vi "editTest.vi"(8 "error in (no error)":errorcluster, 11 "TestInterface in":refnum<class "TestInterface.lvclass">) -> (0 "error out":errorcluster, 3 "TestInterface out":refnum<class "TestInterface.lvclass">)   [LabVIEW 2013, in "TestInterface.lvclass"]
uses:
  Tests/TestInterface/TestInterface.lvclass
panel:
  in  "Cancel Button":bool
  in  "OK Button":bool
  in  "Parameters":string[][](table)
  in  "wait":u32[](array[numeric])
  in  "timings":i32[](array[numeric])
  in  "response":bool[](array[boolean])
  in  "name":string
  in  "Commandlist":string
  in  "Command regex":string[](array[string])
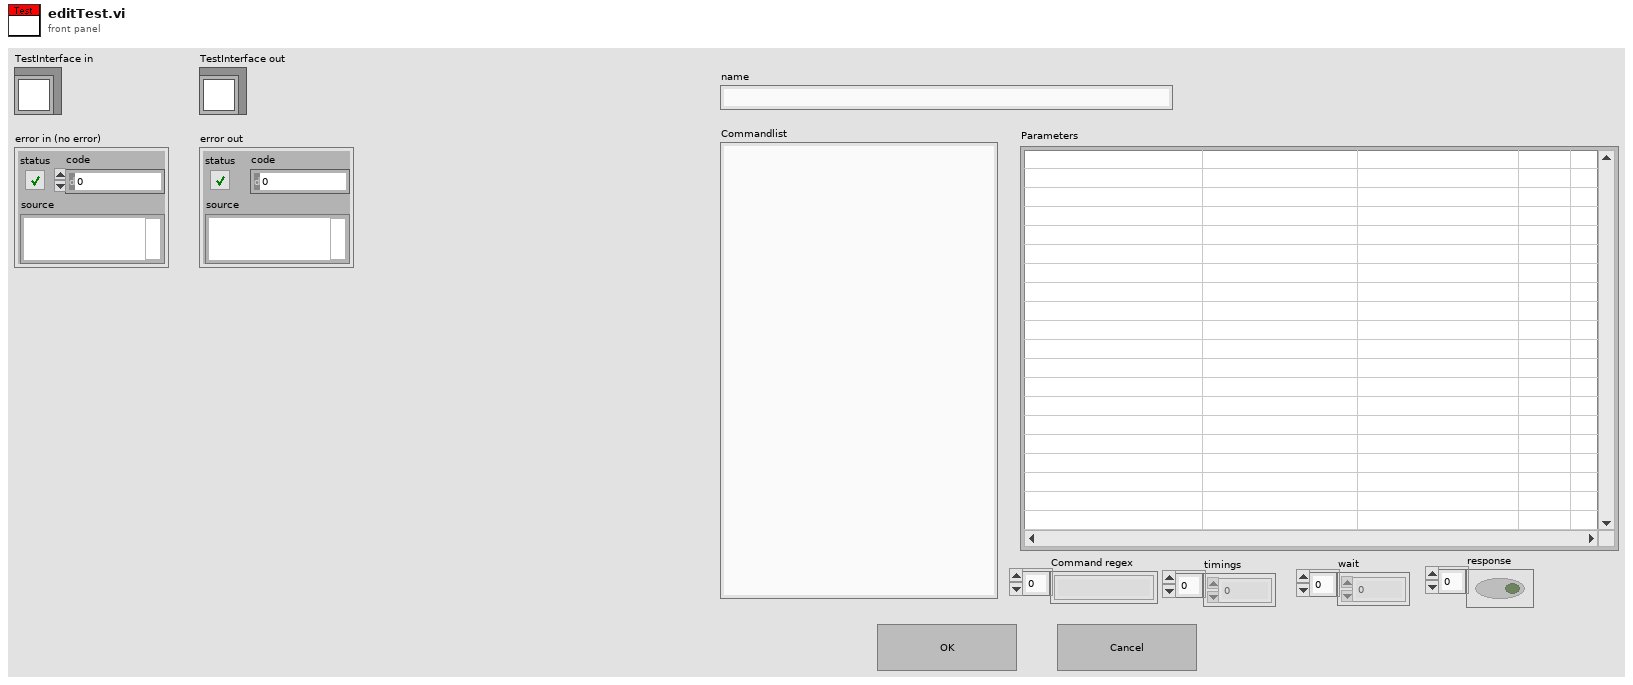
[diagram p1: front panel]
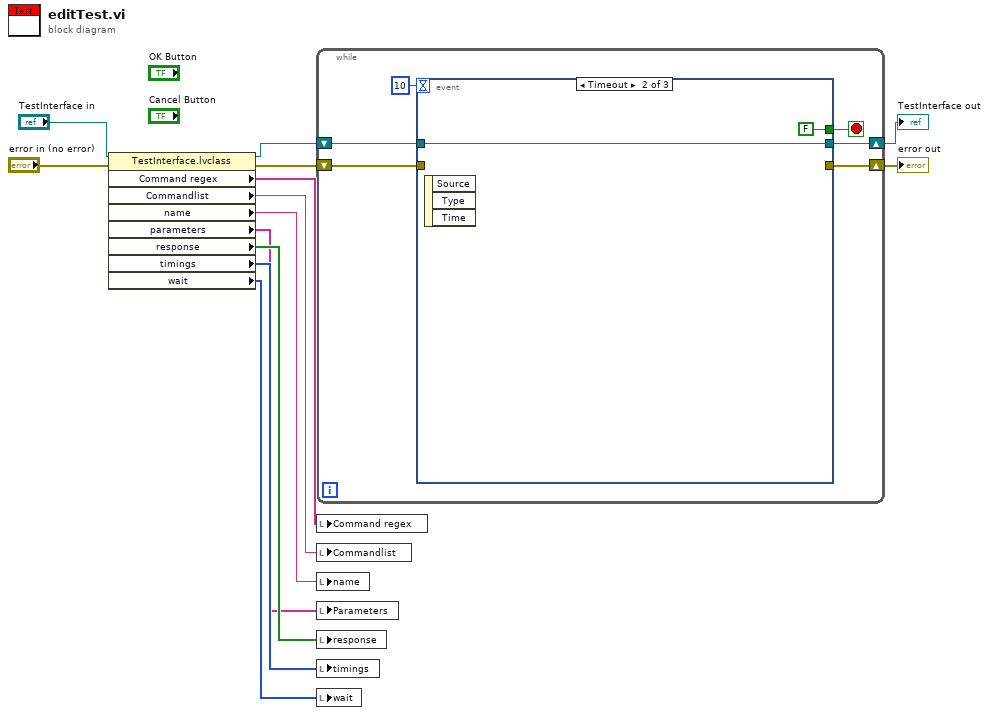
[diagram p0: block diagram]
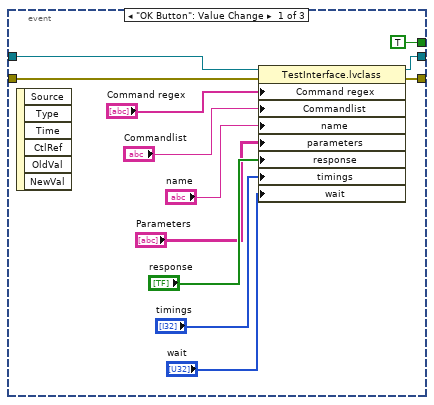
[diagram p2: hidden frame]
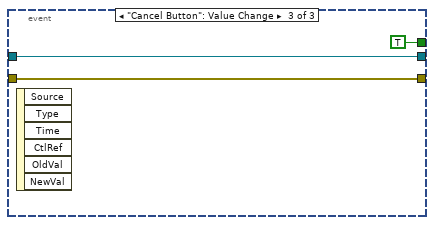
[diagram p3: hidden frame]
diagram:
  n1 = property class="TestInterface.lvclass"(reference="TestInterface in", error in="error in (no error)") -> (reference out=w7:refnum<class "TestInterface.lvclass">, error out=w6:errorcluster, "Command regex"=w13:string[], "Commandlist"=w12:string, "name"=w11:string, "parameters"=w1:string[], "response"=w10:bool[], "timings"=w9:i32[], "wait"=w8:u32[])
  n2 = while {
    shift-right: [w16] -> w4
    shift-left: w7 -> [w19]
    shift-right: [w17] -> w5
    shift-left: w6 -> [w18]
    stop <- w15 stop-if-true
    n3 = event shown="[1] Timeout" {
      selector: _ -> [_ _ _]
      dyn-events: _ -> [_ _ _]
      timeout: 10 -> [_ _ _]
      tunnel: w19 -> [w31 w33 w36]
      tunnel: w18 -> [w30 _ w35]
      tunnel: [w29 _ w35] -> w17
      tunnel: [w28 w33 w36] -> w16
      tunnel: [TRUE FALSE TRUE] -> w15
      event "OK Button": Value Change {
        n4 = event-data() -> ()  [unwired: 1 in, 6 out]
        n5 = property class="TestInterface.lvclass"(reference=w31, error in=w30, "Command regex"="Command regex", "Commandlist"="Commandlist", "name"="name", "parameters"="Parameters", "response"="response", "timings"="timings", "wait"="wait") -> (reference out=w28:refnum<class "TestInterface.lvclass">, error out=w29:errorcluster)
      }
      event Timeout {
        n6 = event-data() -> ()  [unwired: 1 in, 3 out]
      }
      event "Cancel Button": Value Change {
        n7 = event-data() -> ()  [unwired: 1 in, 6 out]
      }
    }
  }
  "error out" <- w5
  "TestInterface out" <- w4
  n8 = local write "Command regex"(w13) -> ()
  n9 = local write "Commandlist"(w12) -> ()
  n10 = local write "name"(w11) -> ()
  n11 = local write "Parameters"(w1) -> ()
  n12 = local write "response"(w10) -> ()
  n13 = local write "timings"(w9) -> ()
  n14 = local write "wait"(w8) -> ()
